vi "Write timing policy.vi"(8 "error in":errorcluster, 10 "timing policy":T1, 11 "Standard Engine Configuration in":refnum<class "Standard Engine Configuration.lvclass">) -> (0 "error out":errorcluster, 3 "Standard Engine Configuration out":refnum<class "Standard Engine Configuration.lvclass">)   [LabVIEW 2013, in "Standard Engine Configuration.lvclass"]
uses:
  Standard Engine Configuration.lvclass
  timing policy.ctl
  Standard Engine Configuration.lvclass/Standard Engine Configuration.ctl
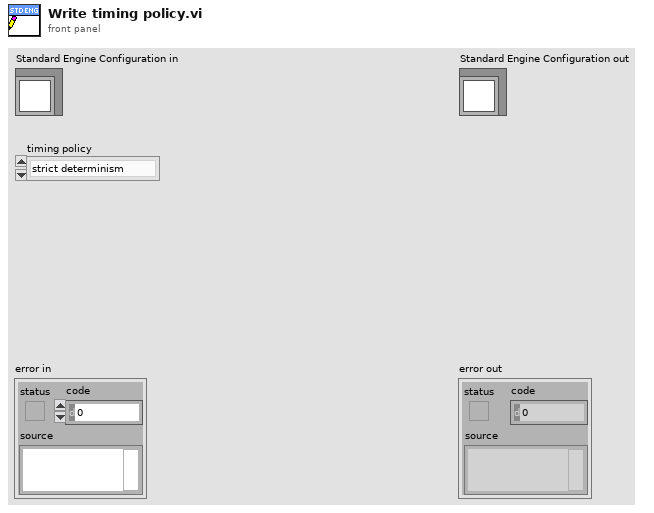
[diagram p1: front panel]
types:
  T1 = typedef "Standard Engine Configuration.lvclass/timing policy.ctl" = enum16{"strict determinism", "nonblocking", "nondeterministic inline"}
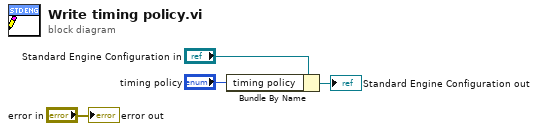
[diagram p0: block diagram]
diagram:
  n1 = Bundle By Name(cluster="Standard Engine Configuration in", "timing policy"="timing policy") -> (→"Standard Engine Configuration out":refnum<class "Standard Engine Configuration.lvclass">)
  "error out" <- "error in"
